vi "Manipulator Daemon.vi"(5 "Manipulator Indicator":T3, 7 "Manipulator Settings":T1, 8 "Error In":errorcluster, 9 "Commands":T2, 11 "VISA resource in":refnum<visa-resource-name>="COM1") -> (0 "Error Out":errorcluster)   [LabVIEW 2012, in "Scientifica Manipulator Daemon.lvlib"]
uses:
  Scientifica Manipulator Daemon.lvlib
  <vilib>/Analysis/Matrix/Datatypes/RealMatrix.ctl
  <vilib>/Analysis/Matrix/NI_Matrix.lvlib
panel:
  out "Abort":bool
  out "Exit":bool
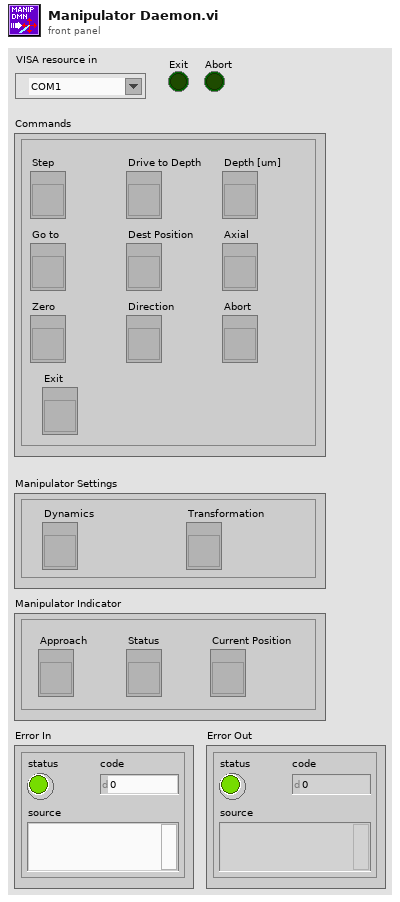
[diagram p1: front panel]
types:
  T1 = cluster{"Dynamics":refnum<vi>, "Transformation":refnum<vi>}
  T2 = cluster{"Zero":refnum<vi>, "Step":refnum<vi>, "Go to":refnum<vi>, "Drive to Depth":refnum<vi>, "Exit":refnum<vi>, "Abort":refnum<vi>, "Depth [um]":refnum<vi>, "Dest Position":refnum<vi>, "Axial":refnum<vi>, "Direction":refnum<vi>}
  T3 = cluster{"Approach":refnum<vi>, "Status":refnum<vi>, "Current Position":refnum<vi>}
  T4 = cluster{"Start speed":i32, "Top Speed":i32, "Acceleration":i32}
  T5 = cluster{"Step length [um]":dbl, "Interstep Interval [ms]":u32, "Initial Speed [um/s]":dbl, "Max Speed [um/s]":dbl, "Acceleration [um/s^2]":dbl, "Max Depth [um]":dbl, "Max Penetration [um]":dbl}
  T6 = typedef "NI_Matrix.lvlib/RealMatrix.ctl" = dbl[][]
  T7 = cluster{"X [um]":dbl, "Y [um]":dbl, "Z [um]":dbl}
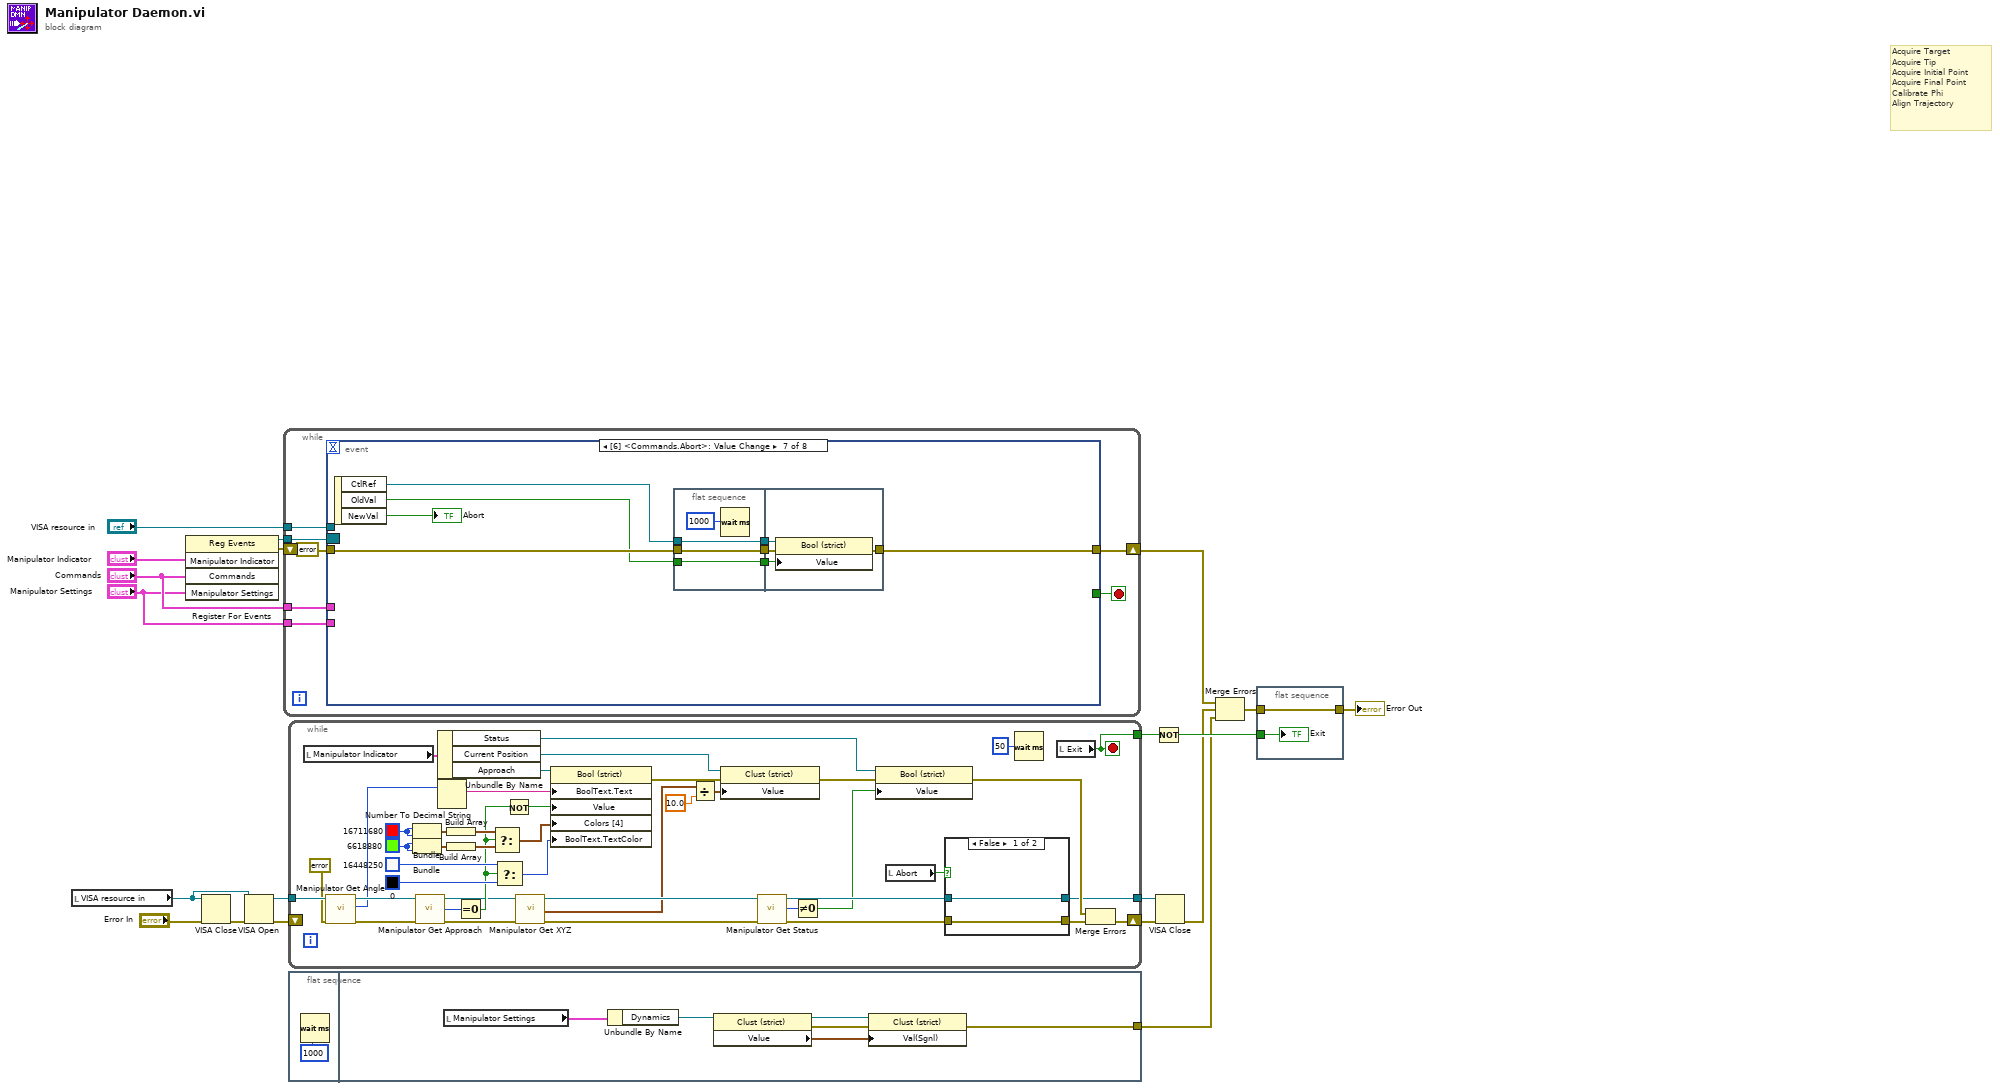
[diagram p0: block diagram]
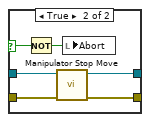
[diagram p2: hidden frame]
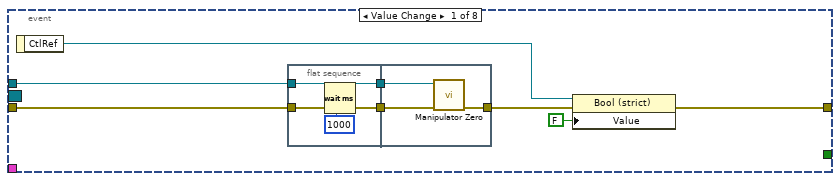
[diagram p3: hidden frame]
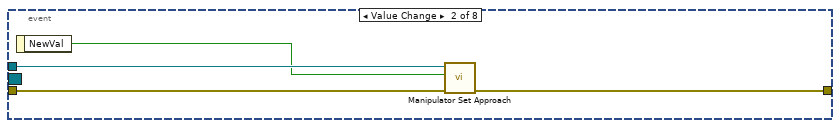
[diagram p4: hidden frame]
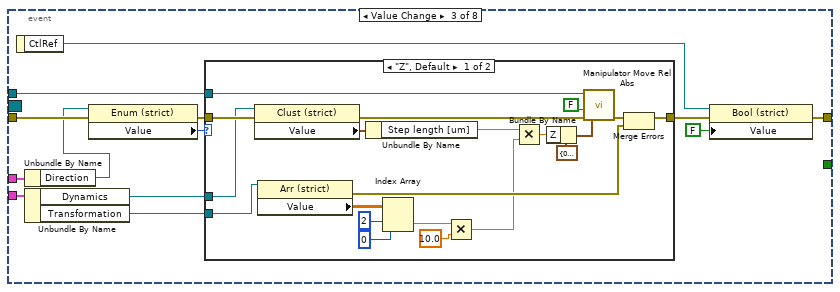
[diagram p5: hidden frame]
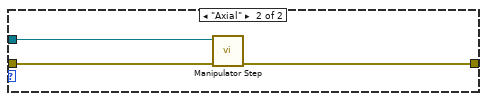
[diagram p6: hidden frame]
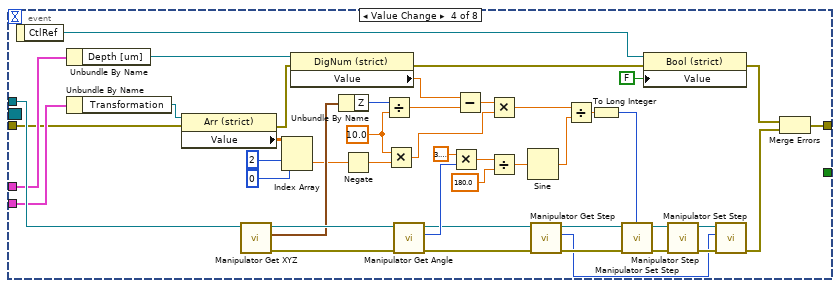
[diagram p7: hidden frame]
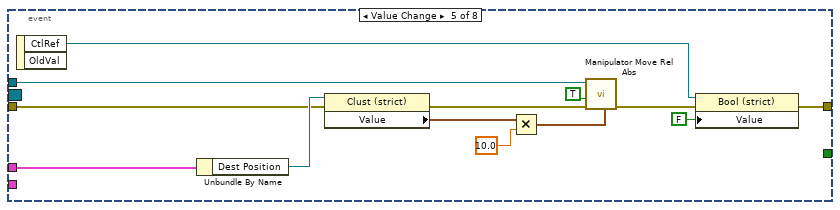
[diagram p8: hidden frame]
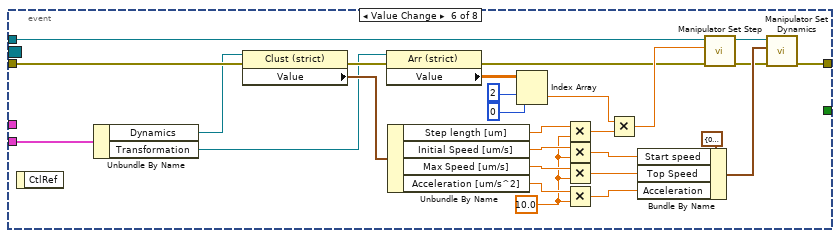
[diagram p9: hidden frame]
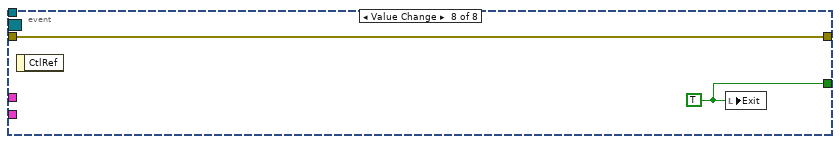
[diagram p10: hidden frame]
diagram:
  # "Acquire Target\nAcquire Tip\nAcquire Initial Point\nAcquire Final Point\nCalibrate Phi\nAlign Trajectory"
  n1 = local read "VISA resource in"() -> (w5:refnum<visa-resource-name>)
  n2 = register-events("Manipulator Indicator", "Commands", "Manipulator Settings") -> (reference out=w11:refnum<event-registration>, error out=w7:errorcluster)  [unwired: 2 in]
  n3 = VISA Close(VISA resource name=w5, error in (no error)="Error In") -> (error out=w18:errorcluster)
  n4 = VISA Open(error in (no error)=w18, VISA resource name=w5) -> (VISA resource name=w20:refnum<visa-resource-name>, error out=w19:errorcluster)  [unwired: 3 in]
  n5 = while {
    tunnel: "VISA resource in" -> [w27]
    shift-right: [w26] -> w4
    shift-left: w7 -> [_]
    tunnel: w11 -> [w24]
    tunnel: "Manipulator Settings" -> [w23]
    tunnel: "Commands" -> [w22]
    stop <- w25 stop-if-true
    n6 = event shown="[6] <Commands.Abort>: Value Change" {
      selector: w24 -> [_ _ _ _ _ _ _ _]
      dyn-events: _ -> [_ _ _ _ _ _ _ _]
      timeout: _ -> [_ _ _ _ _ _ _ _]
      tunnel: w27 -> [w35 w44 w56 w95 w138 w165 _ _]
      tunnel: [_ _ _ _ _ _ _ w183] -> w25
      tunnel: errorcluster {"status"=FALSE, "code"=0, "source"=""} ("error out") -> [w34 w45 w51 w88 w135 w164 w173 w184]
      tunnel: [w32 w42 w55 w87 w129 w159 w172 w184] -> w26
      tunnel: w23 -> [_ _ w50 w90 _ w141 _ _]
      tunnel: w22 -> [_ _ w48 w89 w133 _ _ _]
      event Value Change {
        n7 = event-data() -> ("CtlRef"=w30:refnum<vi>)  [unwired: 1 in]
        n8 = flat-sequence {
          tunnel: w34 -> [w37]
          tunnel: w35 -> [w38]
          tunnel: [w38] -> w29
          tunnel: [w37] -> w28
          tunnel: [w39] -> w31
          tunnel: w29 -> [w41]
          tunnel: w28 -> [w40]
          frame #0 {
            n9 = Wait (ms)(milliseconds to wait=u32 1000) -> ()  [unwired: 1 out]
          }
          frame #1 {
            n10 = call "Manipulator Zero.vi"("error in (no error)"=w40, "VISA resource in"=w41) -> ("error out"=w39:errorcluster)  [unwired: 7 in, 2 out]
          }
        }
        n11 = property class="Bool (strict)"(reference=w30, error in=w31, "Value"=FALSE) -> (error out=w32:errorcluster)  [unwired: 1 out]
      }
      event Value Change {
        n12 = event-data() -> ("NewVal"=w43:bool)  [unwired: 1 in]
        n13 = call "Manipulator Set Approach.vi"("error in (no error)"=w45, "SET/RESET"=w43, "VISA resource in"=w44) -> ("error out"=w42:errorcluster)  [unwired: 6 in, 2 out]
      }
      event Value Change {
        n14 = event-data() -> ("CtlRef"=w57:refnum<vi>)  [unwired: 1 in]
        n15 = Unbundle By Name(w48) -> ("Direction"=w47:refnum<vi>)
        n16 = Unbundle By Name(w50) -> ("Dynamics"=w49:refnum<vi>, "Transformation"=w46:refnum<vi>)
        n17 = property class="Enum (strict)"(reference=w47, error in=w51) -> (error out=w53:errorcluster, "Value"=w52:enum16{"Z", "Axial"})  [unwired: 1 out]
        n18 = case shown="\"Z\", Default" w52 {
          tunnel: [w63 w81] -> w58
          tunnel: w56 -> [w77 w80]
          tunnel: w53 -> [w76 w79]
          tunnel: w49 -> [w75 _]
          tunnel: w46 -> [w65 _]
          frame "Z", Default {
            n19 = property class="Clust (strict)"(reference=w75, error in=w76) -> (error out=w73:errorcluster, "Value"=w74:T5)  [unwired: 1 out]
            n20 = property class="Arr (strict)"(reference=w65) -> (error out=w62:errorcluster, "Value"=w66:T6)  [unwired: 1 in, 1 out]
            n21 = Unbundle By Name(w74) -> ("Step length [um]"=w72:dbl)
            n22 = Index Array(array=w66, index (row)=2, index (col)=0 ("disabled index (col)")) -> (element=w61:dbl)
            n23 = Multiply(x=w61, y=10.0) -> (x*y=w59:dbl)
            n24 = Multiply(x=w72, y=w59) -> (x*y=w70:dbl)
            n25 = Bundle By Name(cluster=cluster{"X":i32, "Y":i32, "Z":i32} {"X"=0, "Y"=0, "Z"=0} ("Deltas"), "Z"=w70) -> (w69:cluster{"X":i32, "Y":i32, "Z":i32})
            n26 = call "Manipulator Move Rel Abs.vi"("error in (no error)"=w73, "ABS"=FALSE, "Deltas"=w69, "VISA resource in"=w77) -> ("error out"=w64:errorcluster)  [unwired: 5 in, 2 out]
            n27 = Merge Errors(w64, w62) -> (w63:errorcluster)
          }
          frame "Axial" {
            n28 = call "Manipulator Step.vi"("error in (no error)"=w79, "VISA resource in"=w80) -> ("error out"=w81:errorcluster)  [unwired: 7 in, 2 out]
          }
        }
        n29 = property class="Bool (strict)"(reference=w57, error in=w58, "Value"=FALSE) -> (error out=w55:errorcluster)  [unwired: 1 out]
      }
      event Value Change {
        w111 = 10.0
        n30 = event-data() -> ("CtlRef"=w83:refnum<vi>)  [unwired: 1 in]
        n31 = Unbundle By Name(w89) -> ("Depth [um]"=w126:refnum<vi>)
        n32 = Unbundle By Name(w90) -> ("Transformation"=w91:refnum<vi>)
        n33 = property class="Arr (strict)"(reference=w91, error in=w88) -> (error out=w92:errorcluster, "Value"=w104:T6)  [unwired: 1 out]
        n34 = call "Manipulator Get XYZ.vi"("VISA resource in"=w95) -> ("error out"=w119:errorcluster, "Coordinates"=w117:cluster{"X":i32, "Y":i32, "Z":i32}, "VISA resource out"=w118:refnum<visa-resource-name>)  [unwired: 8 in]
        n35 = Index Array(array=w104, index (row)=2, index (col)=0 ("disabled index (col)")) -> (element=w105:dbl)
        n36 = property class="DigNum (strict)"(reference=w126, error in=w92) -> (error out=w85:errorcluster, "Value"=w108:dbl)  [unwired: 1 out]
        n37 = Unbundle By Name(w117) -> ("Z"=w115:i32)
        n38 = Negate(x=w105) -> (-x=w109:dbl)
        n39 = Divide(x=w115, y=w111) -> (x/y=w116:dbl)
        n40 = Multiply(x=w111, y=w109) -> (x*y=w110:dbl)
        n41 = call "Manipulator Get Angle.vi"("error in (no error)"=w119, "VISA resource in"=w118) -> ("error out"=w94:errorcluster, "Angle"=w121:i32, "VISA resource out"=w93:refnum<visa-resource-name>)  [unwired: 7 in]
        n42 = Multiply(x=3.141592653589793, y=w121) -> (x*y=w123:dbl)
        n43 = Subtract(x=w108, y=w116) -> (x-y=w114:dbl)
        n44 = Multiply(x=w114, y=w110) -> (x*y=w113:dbl)
        n45 = Divide(x=w123, y=180.0) -> (x/y=w124:dbl)
        n46 = Sine(x=w124) -> (sin(x)=w125:dbl)
        n47 = call "Manipulator Get Step.vi"("error in (no error)"=w94, "VISA resource in"=w93) -> ("error out"=w99:errorcluster, "Step Size"=w96:i32, "VISA resource out"=w100:refnum<visa-resource-name>)  [unwired: 7 in]
        n48 = Divide(x=w113, y=w125) -> (x/y=w112:dbl)
        n49 = To Long Integer(number=w112) -> (32bit integer=w103:i32)
        n50 = call "Manipulator Set Step.vi"("error in (no error)"=w99, "Step"=w103, "VISA resource in"=w100) -> ("error out"=w101:errorcluster, "VISA resource out"=w102:refnum<visa-resource-name>)  [unwired: 6 in, 1 out]
        n51 = property class="Bool (strict)"(reference=w83, error in=w85, "Value"=FALSE) -> (error out=w84:errorcluster)  [unwired: 1 out]
        n52 = call "Manipulator Step.vi"("error in (no error)"=w101, "VISA resource in"=w102) -> ("error out"=w98:errorcluster, "VISA resource out"=w97:refnum<visa-resource-name>)  [unwired: 7 in, 1 out]
        n53 = call "Manipulator Set Step.vi"("error in (no error)"=w98, "Step"=w96, "VISA resource in"=w97) -> ("error out"=w86:errorcluster)  [unwired: 6 in, 2 out]
        n54 = Merge Errors(w84, w86) -> (w87:errorcluster)
      }
      event Value Change {
        n55 = event-data() -> ("CtlRef"=w128:refnum<vi>)  [unwired: 1 in, 1 out]
        n56 = Unbundle By Name(w133) -> ("Dest Position"=w139:refnum<vi>)
        n57 = property class="Clust (strict)"(reference=w139, error in=w135) -> (error out=w136:errorcluster, "Value"=w132:T7)  [unwired: 1 out]
        n58 = Multiply(x=w132, y=10.0) -> (x*y=w134:T7)
        n59 = call "Manipulator Move Rel Abs.vi"("error in (no error)"=w136, "ABS"=TRUE, "Deltas"=w134, "VISA resource in"=w138) -> ("error out"=w130:errorcluster)  [unwired: 5 in, 2 out]
        n60 = property class="Bool (strict)"(reference=w128, error in=w130, "Value"=FALSE) -> (error out=w129:errorcluster)  [unwired: 1 out]
      }
      event Value Change {
        w154 = 10.0 ("y")
        n61 = event-data() -> ()  [unwired: 1 in, 1 out]
        n62 = Unbundle By Name(w141) -> ("Dynamics"=w142:refnum<vi>, "Transformation"=w140:refnum<vi>)
        n63 = property class="Clust (strict)"(reference=w142, error in=w164) -> (error out=w148:errorcluster, "Value"=w166:T5)  [unwired: 1 out]
        n64 = property class="Arr (strict)"(reference=w140, error in=w148) -> (error out=w147:errorcluster, "Value"=w146:T6)  [unwired: 1 out]
        n65 = Unbundle By Name(w166) -> ("Step length [um]"=w163:dbl, "Initial Speed [um/s]"=w157:dbl, "Max Speed [um/s]"=w156:dbl, "Acceleration [um/s^2]"=w155:dbl)
        n66 = Index Array(array=w146, index (row)=2, index (col)=0 ("disabled index (col)")) -> (element=w143:dbl)
        n67 = Multiply(x=w163, y=w154) -> (x*y=w150:dbl)
        n68 = Multiply(x=w157, y=w154) -> (x*y=w153:dbl)
        n69 = Multiply(x=w156, y=w154) -> (x*y=w152:dbl)
        n70 = Multiply(x=w155, y=w154) -> (x*y=w151:dbl)
        n71 = Multiply(x=w143, y=w150) -> (x*y=w149:dbl)
        n72 = Bundle By Name(cluster=T4 {"Start speed"=0, "Top Speed"=0, "Acceleration"=0} ("Inputs"), "Start speed"=w153, "Top Speed"=w152, "Acceleration"=w151) -> (w162:T4)
        n73 = call "Manipulator Set Step.vi"("error in (no error)"=w147, "Step"=w149, "VISA resource in"=w165) -> ("error out"=w160:errorcluster, "VISA resource out"=w158:refnum<visa-resource-name>)  [unwired: 6 in, 1 out]
        n74 = call "Manipulator Set Dynamics.vi"("error in (no error)"=w160, "Inputs"=w162, "VISA resource in"=w158) -> ("error out"=w159:errorcluster)  [unwired: 6 in, 2 out]
      }
      event Value Change {
        n75 = event-data() -> ("CtlRef"=w171:refnum<vi>, "OldVal"=w170:bool, "NewVal"=→"Abort":bool)  [unwired: 1 in]
        n76 = flat-sequence {
          tunnel: w170 -> [w176]
          tunnel: w171 -> [w177]
          tunnel: w173 -> [w178]
          tunnel: [w178] -> w169
          tunnel: [w177] -> w168
          tunnel: [w176] -> w167
          tunnel: [w181] -> w172
          tunnel: w169 -> [w182]
          tunnel: w168 -> [w180]
          tunnel: w167 -> [w179]
          frame #0 {
            n77 = Wait (ms)(milliseconds to wait=u32 1000) -> ()  [unwired: 1 out]
          }
          frame #1 {
            n78 = property class="Bool (strict)"(reference=w180, error in=w182, "Value"=w179) -> (error out=w181:errorcluster)  [unwired: 1 out]
          }
        }
      }
      event Value Change {
        w183 = TRUE ("NewVal")
        n79 = event-data() -> ()  [unwired: 1 in, 1 out]
        n80 = local write "Exit"(w183) -> ()
      }
    }
  }
  n81 = while {
    tunnel: w20 -> [w226]
    shift-right: [w196] -> w13
    shift-left: w19 -> [_]
    tunnel: [w217] -> w12
    tunnel: [w193] -> w2
    stop <- w217 stop-if-true
    w216 = u32 6618880
    w215 = u32 16711680
    n82 = local read "Manipulator Indicator"() -> (w209:T3)
    n83 = call "Manipulator Get Angle.vi"("error in (no error)"=errorcluster {"status"=FALSE, "code"=0, "source"=""} ("error out"), "VISA resource in"=w226) -> ("error out"=w222:errorcluster, "Angle"=w219:i32, "VISA resource out"=w223:refnum<visa-resource-name>)  [unwired: 7 in]
    n84 = Bundle(w215, w215) -> (w214:cluster{u32, u32})  [unwired: 1 in]
    n85 = Bundle(w216, w216) -> (w212:cluster{u32, u32})  [unwired: 1 in]
    n86 = call "Manipulator Get Approach.vi"("error in (no error)"=w222, "VISA resource in"=w223) -> ("error out"=w208:errorcluster, "Response"=w220:i32, "VISA resource out"=w206:refnum<visa-resource-name>)  [unwired: 7 in]
    n87 = Unbundle By Name(w209) -> ("Status"=w200:refnum<vi>, "Current Position"=w227:refnum<vi>, "Approach"=w199:refnum<vi>)
    n88 = Number To Decimal String(number=w219) -> (decimal integer string=w192:string)  [unwired: 1 in]
    n89 = Build Array(w214) -> (w213:cluster{u32, u32}[])
    n90 = Build Array(w212) -> (w211:cluster{u32, u32}[])
    n91 = Equal To 0?(x=w220) -> (x = 0?=w210:bool)
    n92 = Select(t=w213, s=w210, f=w211) -> (s? t:f=w203:cluster{u32, u32}[])
    n93 = Select(t=u32 16448250, s=w210, f=u32 0) -> (s? t:f=w202:u32)
    n94 = Not(x=w210) -> (.not. x?=w204:bool)
    n95 = call "Manipulator Get XYZ.vi"("error in (no error)"=w208, "VISA resource in"=w206) -> ("error out"=w207:errorcluster, "Coordinates"=w187:cluster{"X":i32, "Y":i32, "Z":i32}, "VISA resource out"=w205:refnum<visa-resource-name>)  [unwired: 7 in]
    n96 = property class="Bool (strict)"(reference=w199, "BoolText.Text"=w192, "Value"=w204, "Colors [4]"=w203, "BoolText.TextColor"=w202) -> (error out=w218:errorcluster)  [unwired: 1 in, 1 out]
    n97 = Divide(x=w187, y=10.0) -> (x/y=w188:cluster{"X":dbl, "Y":dbl, "Z":dbl})
    n98 = property class="Clust (strict)"(reference=w227, error in=w218, "Value"=w188) -> (error out=w201:errorcluster)  [unwired: 1 out]
    n99 = call "Manipulator Get Status.vi"("error in (no error)"=w207, "VISA resource in"=w205) -> ("error out"=w191:errorcluster, "Status"=w221:i32, "VISA resource out"=w198:refnum<visa-resource-name>)  [unwired: 7 in]
    n100 = Not Equal To 0?(x=w221) -> (x != 0?=w197:bool)
    n101 = property class="Bool (strict)"(reference=w200, error in=w201, "Value"=w197) -> (error out=w194:errorcluster)  [unwired: 1 out]
    n102 = local read "Abort"() -> (w190:bool)
    n103 = case shown="False" w190 {
      selector: w190 -> [_ w231]
      tunnel: w198 -> [w229 w235]
      tunnel: [w229 w234] -> w193
      tunnel: [w228 w233] -> w195
      tunnel: w191 -> [w228 w232]
      frame False {
      }
      frame True {
        n104 = Not(x=w231) -> (.not. x?=w230:bool)
        n105 = call "Manipulator Stop Move.vi"("error in (no error)"=w232, "VISA resource in"=w235) -> ("error out"=w233:errorcluster, "VISA resource out"=w234:refnum<visa-resource-name>)  [unwired: 7 in, 1 out]
        n106 = local write "Abort"(w230) -> ()
      }
    }
    n107 = Wait (ms)(milliseconds to wait=u32 50) -> ()  [unwired: 1 out]
    n108 = local read "Exit"() -> (w217:bool)
    n109 = Merge Errors(w194, w195) -> (w196:errorcluster)
  }
  n110 = flat-sequence {
    tunnel: [w237] -> w1
    frame #0 {
      n111 = Wait (ms)(milliseconds to wait=u32 1000) -> ()  [unwired: 1 out]
    }
    frame #1 {
      n112 = local read "Manipulator Settings"() -> (w238:T1)
      n113 = Unbundle By Name(w238) -> ("Dynamics"=w239:refnum<vi>)
      n114 = property class="Clust (strict)"(reference=w239) -> (reference out=w242:refnum<vi>, error out=w241:errorcluster, "Value"=w240:T5)  [unwired: 1 in]
      n115 = property class="Clust (strict)"(reference=w242, error in=w241, "Val(Sgnl)"=w240) -> (error out=w237:errorcluster)  [unwired: 1 out]
    }
  }
  n116 = Not(x=w12) -> (.not. x?=w14:bool)
  n117 = VISA Close(VISA resource name=w2, error in (no error)=w13) -> (error out=w3:errorcluster)
  n118 = Merge Errors(w4, w3, w1) -> (w15:errorcluster)
  n119 = flat-sequence {
    tunnel: [w244] -> w16
    tunnel: w15 -> [w244]
    tunnel: w14 -> [w243]
    frame #0 {
      "Exit" <- w243
    }
  }
  "Error Out" <- w16
